vi "Questao2VF_Ulisses.vi"() -> ()   [LabVIEW 2019]
uses:
  <vilib>/measure/matone.llb/Extract Single Tone Information 1 Chan.vi
  <vilib>/measure/NI_MAPro.lvlib
panel:
  in  "Path":path
  out "Y max":dbl format="%0.2f"
  out "Waveform Graph 2":dbl[](graph)
  out "detected frequency":dbl format="%.2p"
  out "detected amplitude":dbl format="%.2p"
  out "dt":dbl
  out "size(s)":i32
  out "Sinal completo":waveform(dbl)(graph)
  # "Phase em graus"
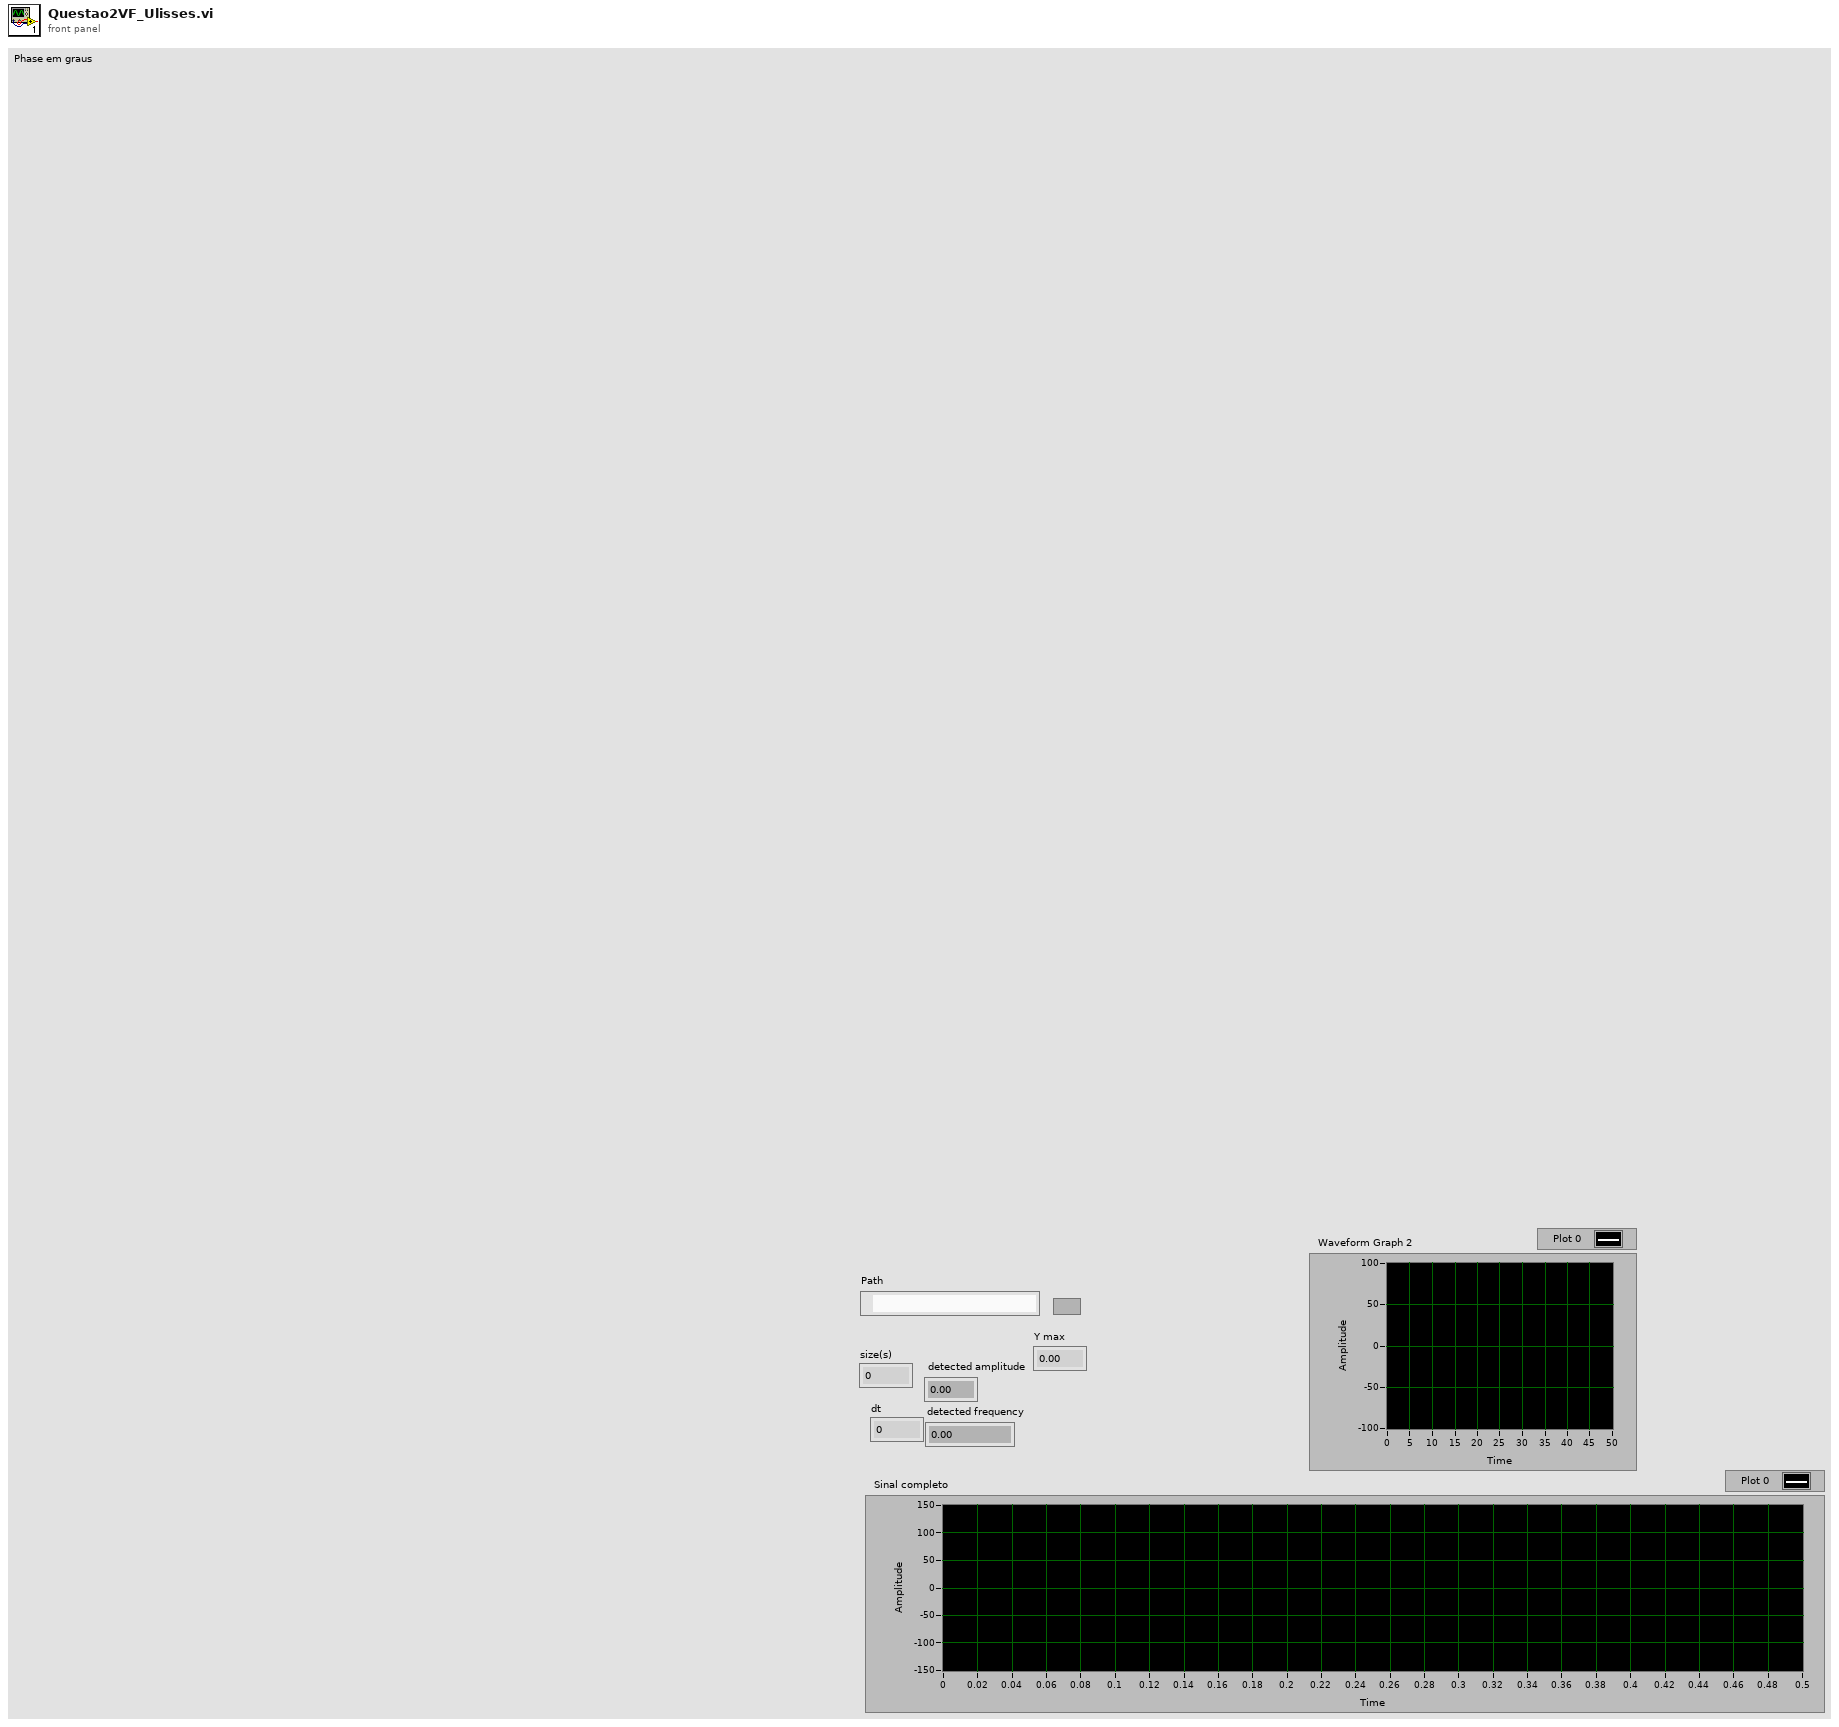
[diagram p1: front panel]
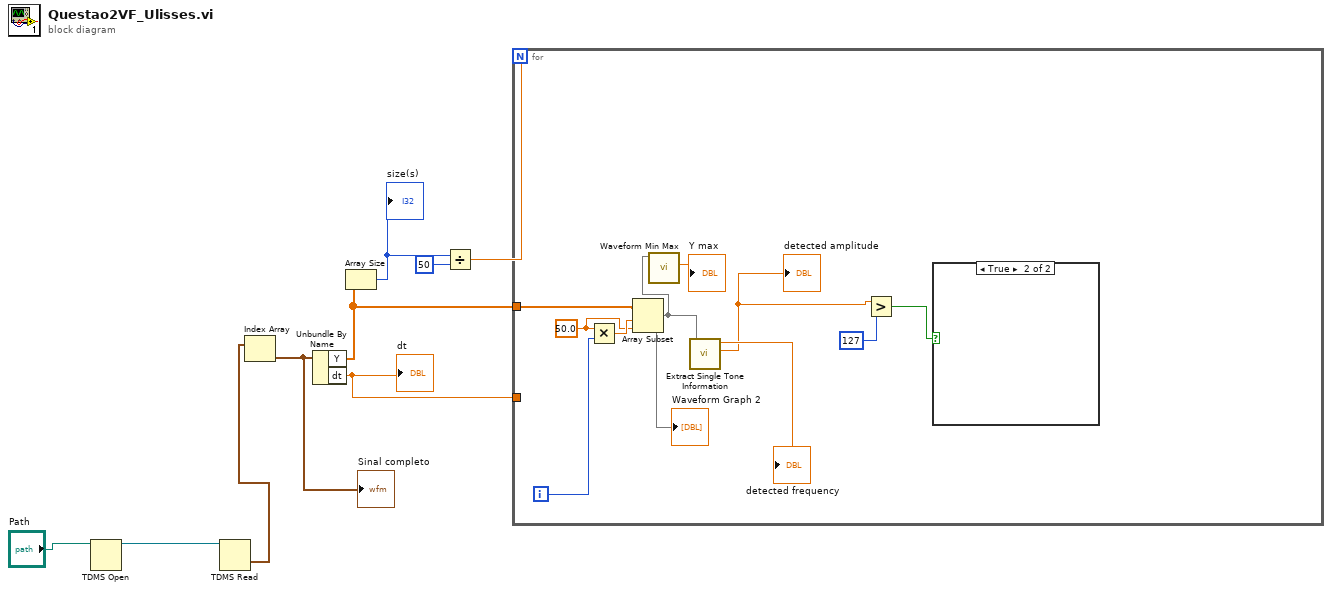
[diagram p0: block diagram]
diagram:
  n1 = TDMS Open(11:"Path") -> (3:w9:refnum<k34>)  [unwired: 6 in, 1 out]
  n2 = TDMS Read(0:w9) -> (10:w8:waveform(dbl)[])  [unwired: 7 in, 5 out]
  n3 = Index Array(array=w8) -> (element=w7:waveform(dbl))  [unwired: 1 in]
  "Sinal completo" <- w7
  n4 = Unbundle By Name(w7) -> ("Y"=w3:dbl[], "dt"=w4:dbl)
  "dt" <- w4
  n5 = Array Size(array=w3) -> (size(s)=w6:i32)
  "size(s)" <- w6
  n6 = Divide(x=w6, y=50) -> (x/y=w1:dbl)
  n7 = for {
    N: w1 -> [_]
    tunnel: w3 -> [w19]
    tunnel: w4 -> [_]
    i -> [w18]
    w16 = 50.0 ("x")
    n8 = Multiply(x=w16, y=w18) -> (x*y=w17:dbl)
    n9 = Array Subset(array=w19, index=w17, length=w16) -> (w13:dbl[])
    "Waveform Graph 2" <- w13
    n10 = call <vilib>:"Waveform Min Max.vi"("waveform in"=w13) -> ("Y max"=→"Y max":dbl)  [unwired: 5 in, 5 out]
    n11 = call-poly <vilib>:"Extract Single Tone Information.vi"("time signal in"=w13) -> ("detected amplitude"=w12:dbl, "detected frequency"=→"detected frequency":dbl)  [unwired: 5 in, 4 out]
    "detected amplitude" <- w12
    n12 = Greater?(x=w12, y=127) -> (0:w10:bool)
    n13 = case shown="True" w10 {
      frame False {
      }
      frame True {
      }
    }
  }
